vi "Change_Enum.vi"() -> ()   [LabVIEW 2013]
panel:
  out "error out":errorcluster
  in  "Strings []":string[](array[string])=["This", "is", "after"]
  in  "target class":refnum<vi>
  in  "vi path":path=path "enum_target.vi"
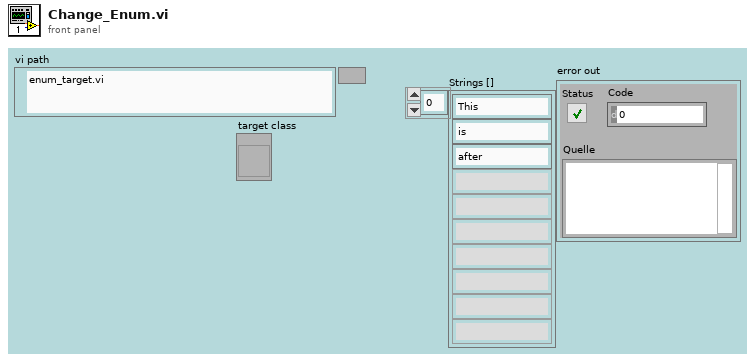
[diagram p1: front panel]
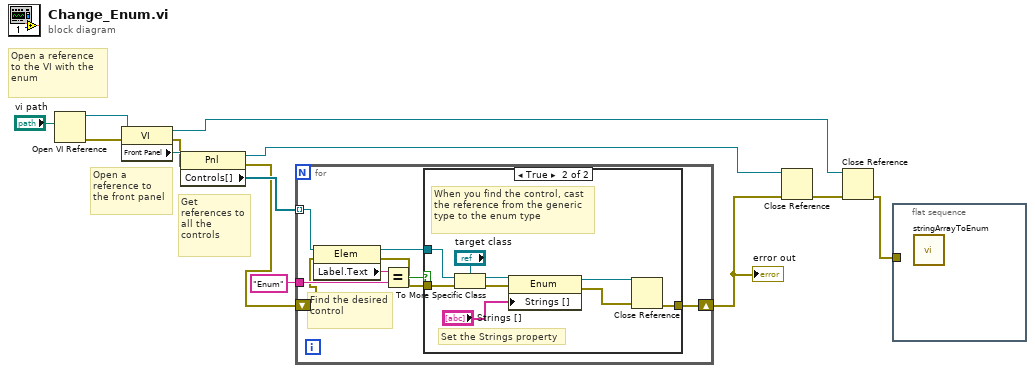
[diagram p0: block diagram]
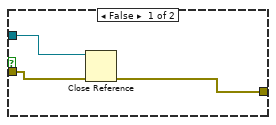
[diagram p2: hidden frame]
diagram:
  # "Open a reference to the VI with the enum"
  # "Open a reference to the front panel"
  # "Get references to all the controls"
  n1 = Open VI Reference(vi path="vi path") -> (vi reference=w13:refnum<vi>, error out=w6:errorcluster)  [unwired: 5 in]
  n2 = property class="VI"(reference=w13, error in=w6) -> (reference out=w10:refnum<vi>, error out=w5:errorcluster, "Front Panel"=w12:refnum<vi>)
  n3 = property class="Pnl"(reference=w12, error in=w5) -> (reference out=w9:refnum<vi>, error out=w4:errorcluster, "Controls[]"=w8:refnum<vi>[])
  n4 = for {
    tunnel: w8 -> [w21] mode=indexing
    tunnel: "Enum" -> [w19]
    shift-right: [w14] -> w3
    shift-left: w4 -> [w16]
    # "Find the desired control"
    n5 = property class="Elem"(reference=w21, error in=w16) -> (reference out=w17:refnum<vi>, error out=w15:errorcluster, "Label.Text"=w20:string)
    n6 = Equal?(x=w20, y=w19) -> (x = y?=w18:bool)
    n7 = case shown="True" w18 {
      tunnel: w17 -> [w24 w33]
      tunnel: w15 -> [w23 w28]
      tunnel: [w22 w25] -> w14
      frame False {
        n8 = Close Reference(reference=w24, error in (no error)=w23) -> (error out=w22:errorcluster)
      }
      frame True {
        # "Set the Strings property"
        # "When you find the control, cast the reference from the generic type to the enum type"
        n9 = To More Specific Class(target class="target class", reference=w33, error in=w28) -> (specific class reference=w31:refnum<vi>, error out=w27:errorcluster)
        n10 = property class="Enum"(reference=w31, error in=w27, "Strings []"="Strings []") -> (reference out=w30:refnum<vi>, error out=w26:errorcluster)
        n11 = Close Reference(reference=w30, error in (no error)=w26) -> (error out=w25:errorcluster)
      }
    }
  }
  "error out" <- w3
  n12 = Close Reference(reference=w9, error in (no error)=w3) -> (error out=w2:errorcluster)
  n13 = Close Reference(reference=w10, error in (no error)=w2) -> (error out=w1:errorcluster)
  n14 = flat-sequence {
    tunnel: [w34] -> _
    tunnel: w1 -> [w34]
    frame #0 {
      n15 = call "stringArrayToEnum.vi"() -> ()  [unwired: 12 in]
    }
  }
